vi "Write Device info parameters Ini file.vi"(7 "Instrument info":string[][](array[string]), 8 "Error In":errorcluster, 11 "Start path":path) -> (0 "Error Out":errorcluster)   [LabVIEW 2020, in "Test Framework.lvclass"]
uses:
  Test Framework.lvclass
  <vilib>/Utility/config.llb/Write Key (String).vi
  <vilib>/Utility/config.llb/NI_LVConfig.lvlib
panel:
  out "Cancelled":bool
  in  "Sections to write":string[](array[string])=["User", "Fetched"]
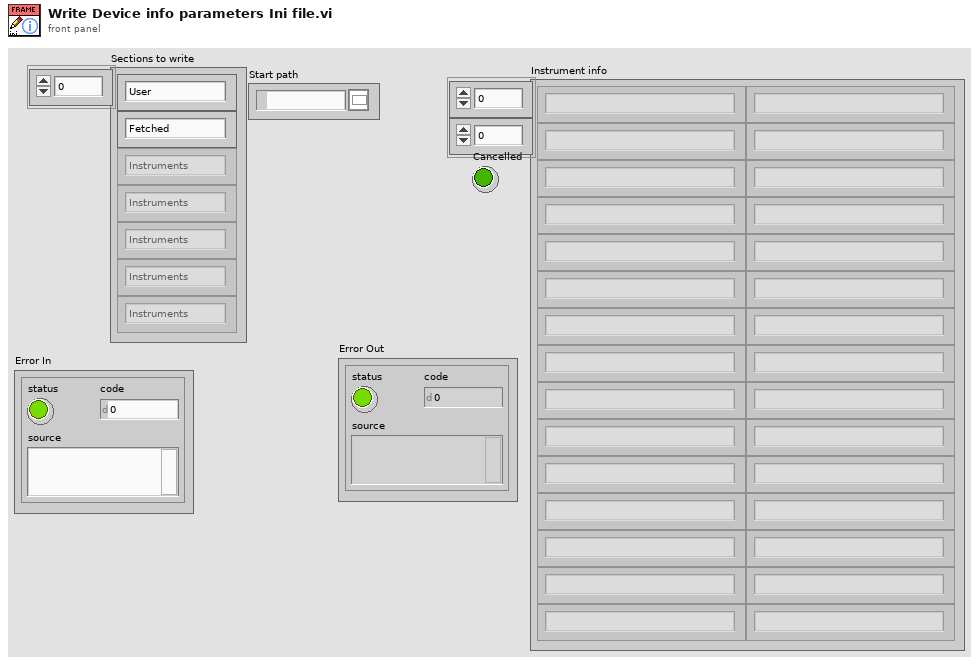
[diagram p1: front panel]
types:
  T1 = typedef "NI_LVConfig.lvlib/Config Data RefNum.ctl" = refnum<k1>
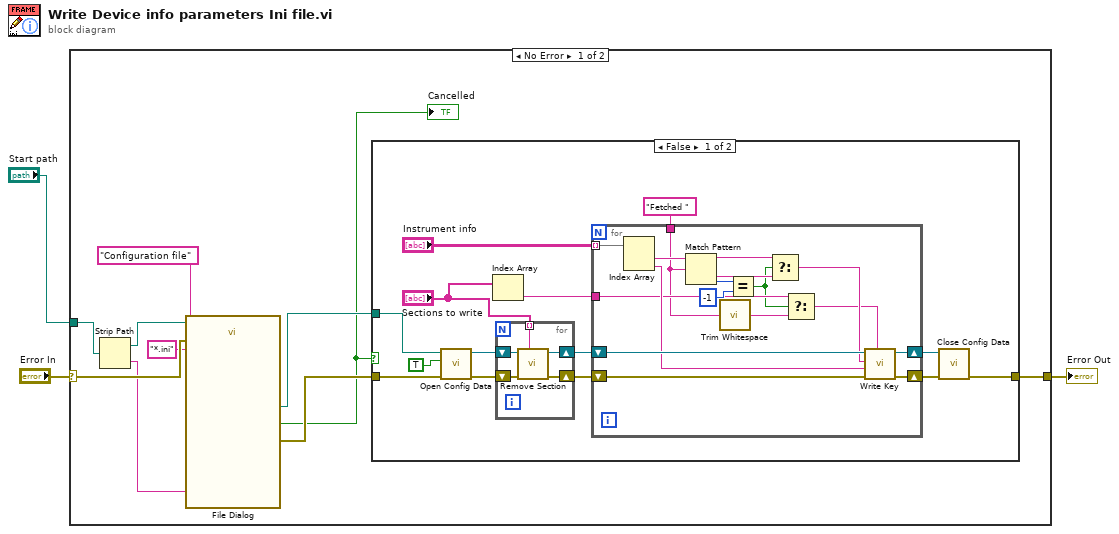
[diagram p0: block diagram]
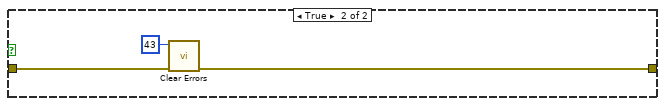
[diagram p2: hidden frame]
diagram:
  n1 = case shown="No Error" "Error In" {
    selector: "Error In" -> [w11 w53]
    tunnel: [w12 w53] -> w2
    tunnel: "Start path" -> [w6 _]
    frame No Error {
      n2 = Strip Path(path=w6) -> (stripped path=w5:path, name=w4:string)
      n3 = call "File Dialog"("start path"=w5, "default name"=w4, "error in"=w11, "pattern (all files)"="*.ini", "pattern label"="Configuration file") -> ("selected path"=w13:path, "cancelled"=w9:bool, "error out"=w10:errorcluster)  [unwired: 7 in, 1 out]
      "Cancelled" <- w9
      n4 = case shown="False" w9 {
        tunnel: w13 -> [w27 _]
        tunnel: [w25 w51] -> w12
        tunnel: w10 -> [w18 w52]
        frame False {
          n5 = call <vilib>:"Open Config Data.vi"("error in (no error)"=w18, "create file if necessary (T)"=TRUE, "configuration file path"=w27) -> ("error out"=w23:errorcluster, "refnum"=w22:T1)  [unwired: 6 in, 1 out]
          n6 = Index Array(array="Sections to write") -> (element=w17:string)  [unwired: 1 in]
          n7 = for {
            tunnel: "Sections to write" -> [w28] mode=indexing
            shift-right: [w29] -> w20
            shift-left: w23 -> [w32]
            shift-right: [w30] -> w21
            shift-left: w22 -> [w31]
            n8 = call <vilib>:"Remove Section.vi"("section"=w28, "error in (no error)"=w32, "refnum"=w31) -> ("error out"=w29:errorcluster, "refnum out"=w30:T1)  [unwired: 6 in, 1 out]
          }
          n9 = for {
            tunnel: w17 -> [w37]
            shift-right: [w45] -> w26
            shift-left: w20 -> [w49]
            shift-right: [w44] -> w24
            shift-left: w21 -> [w48]
            tunnel: "Instrument info" -> [w47] mode=indexing
            tunnel: "Fetched " ("regular expression") -> [w33]
            n10 = Index Array(array=w47) -> (element #1=w39:string, element #2=w46:string)  [unwired: 2 in]
            n11 = Match Pattern(string=w39, regular expression=w33) -> (before substring=w41:string, after substring=w40:string, offset past match=w43:i32)  [unwired: 1 in, 1 out]
            n12 = call <vilib>:"Trim Whitespace.vi"("string"=w33) -> ("trimmed string"=w35:string)  [unwired: 1 in]
            n13 = Equal?(x=w43, y=-1) -> (x = y?=w36:bool)
            n14 = Select(t=w41, s=w36, f=w40) -> (s? t:f=w38:string)
            n15 = Select(t=w37, s=w36, f=w35) -> (s? t:f=w34:string)
            n16 = call-poly <vilib>:"Write Key.vi"("section"=w34, "error in (no error)"=w49, "value"=w46, "key"=w38, "refnum"=w48) -> ("error out"=w45:errorcluster, "refnum out"=w44:T1)  [unwired: 4 in, 1 out]
          }
          n17 = call <vilib>:"Close Config Data.vi"("error in (no error)"=w26, "refnum"=w24) -> ("error out"=w25:errorcluster)  [unwired: 8 in, 1 out]
        }
        frame True {
          n18 = call <vilib>:"Clear Errors.vi"("error in (no error)"=w52, "specific error code to clear (0: all)"=43) -> ("error out"=w51:errorcluster)  [unwired: 4 in, 1 out]
        }
      }
    }
    frame Error {
    }
  }
  "Error Out" <- w2
